vi "1_10.vi"() -> ()   [LabVIEW 2020]
panel:
  out "Second root":string
  out "First root":string
  in  "C":dbl
  in  "B":dbl
  in  "A":dbl
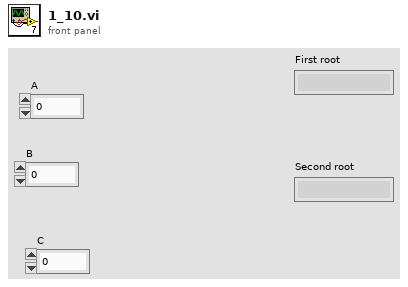
[diagram p1: front panel]
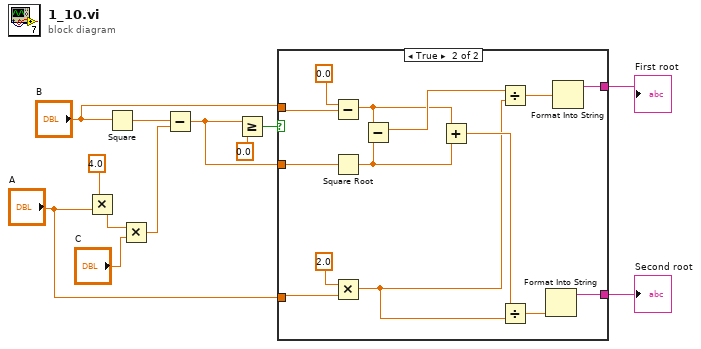
[diagram p0: block diagram]
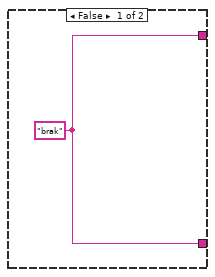
[diagram p2: hidden frame]
diagram:
  n1 = Multiply(x=4.0 ("x*y"), y="A") -> (x*y=w11:dbl)
  n2 = Square(x="B") -> (x^2=w9:dbl)
  n3 = Multiply(x=w11, y="C") -> (x*y=w8:dbl)
  n4 = Subtract(x=w9, y=w8) -> (x-y=w4:dbl)
  n5 = Greater Or Equal?(x=w4, y=0.0) -> (x >= y?=w6:bool)
  n6 = case shown="True" w6 {
    tunnel: "B" -> [_ w26]
    tunnel: w4 -> [_ w25]
    tunnel: "A" -> [_ w23]
    tunnel: [w13 w21] -> w1
    tunnel: [w13 w15] -> w2
    frame False {
      w13 = "brak"
    }
    frame True {
      n7 = Subtract(x=0.0 ("y"), y=w26) -> (x-y=w20:dbl)
      n8 = Square Root(x=w25) -> (sqrt(x)=w19:dbl)
      n9 = Multiply(x=2.0, y=w23) -> (x*y=w17:dbl)
      n10 = Subtract(x=w20, y=w19) -> (x-y=w24:dbl)
      n11 = Add(x=w20, y=w19) -> (x+y=w18:dbl)
      n12 = Divide(x=w24, y=w17) -> (x/y=w22:dbl)
      n13 = Divide(x=w18, y=w17) -> (x/y=w16:dbl)
      n14 = Format Into String(w16) -> (resulting string=w15:string)  [unwired: 3 in, 1 out]
      n15 = Format Into String(w22) -> (resulting string=w21:string)  [unwired: 3 in, 1 out]
    }
  }
  "First root" <- w1
  "Second root" <- w2
